vi "Make VI Param(Read Storage Rsp).vi"(1 "pRsp":T1) -> (0 "Read Storage Rsp":T2)   [LabVIEW 8.6, in "Keyence LJ-V7000.lvlib"]
uses:
  Keyence LJ-V7000.lvlib
  Public/Clusters/Time.ctl
  Public/Clusters/Read Storage Rsp.ctl
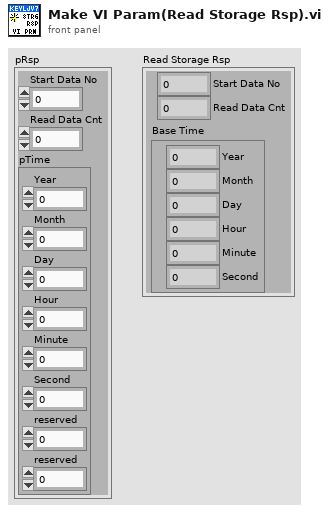
[diagram p1: front panel]
types:
  T1 = cluster{"Start Data No":u32, "Read Data Cnt":u32, "pTime":cluster{"Year":u8, "Month":u8, "Day":u8, "Hour":u8, "Minute":u8, "Second":u8, "reserved":u8, "reserved":u8}}
  T2 = typedef "Keyence LJ-V7000.lvlib/Read Storage Rsp.ctl" = cluster{"Start Data No":u32, "Read Data Cnt":u32, "Base Time":T3}
  T3 = typedef "Keyence LJ-V7000.lvlib/Time.ctl" = cluster{"Year":u8, "Month":u8, "Day":u8, "Hour":u8, "Minute":u8, "Second":u8}
  T4 = cluster{"Year":u8, "Month":u8, "Day":u8, "Hour":u8, "Minute":u8, "Second":u8, "reserved":u8, "reserved":u8}
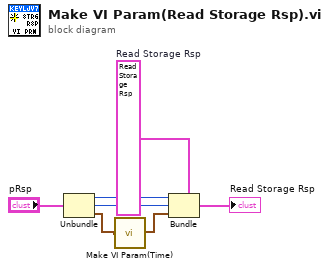
[diagram p0: block diagram]
diagram:
  w6 = T2 ?  # Read Storage Rsp
  n1 = Unbundle("pRsp") -> ("Start Data No"=w2:u32, "Read Data Cnt"=w3:u32, "pTime"=w4:T4)
  n2 = call "Make VI Param(Time).vi"("pTime"=w4) -> ("Time"=w5:T3)
  n3 = Bundle(cluster=w6, "Start Data No"=w2, "Read Data Cnt"=w3, "Base Time"=w5) -> (→"Read Storage Rsp":T2)
